vi "Initialize List Type.vi"(8 "error in (no error)":errorcluster, 11 "Numeric Data Type in":refnum<class "Numeric Data Type.lvclass">) -> (0 "error out":errorcluster, 3 "Numeric Data Type (dup)":refnum<class "Numeric Data Type.lvclass">)   [LabVIEW 2018, in "Numeric Data Type.lvclass"]
uses:
  Numeric Data Type.lvclass
  <vilib>/Utility/miscctls.llb/LVRowAndColumnUnsignedTypeDef.ctl
  Numeric Data Type.lvclass/Numeric Data Type.ctl
  Format Code Type List Enum.ctl
  Reference List Type.vi
  Reference Format Codes.vi
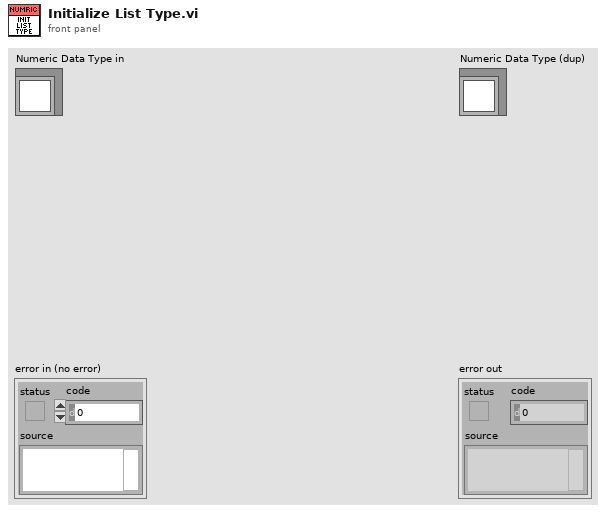
[diagram p1: front panel]
types:
  T1 = typedef "LVRowAndColumnUnsignedTypeDef.ctl" = cluster{"Row":u32, "Column":u32}
  T2 = typedef "Numeric Data Type.lvclass/Format Code Type List Enum.ctl" = enum16{"Numeric format codes", "Relative time format codes", "Absolute time format codes"}
  T3 = typedef "Numeric Data Type.lvclass/Time Info.ctl" = cluster{"Time Format":T4, "Numeric Format":T5, "Clock Type":T6, "Include Seconds?":bool, "Seconds Precision":i16, "Date Order":T7, "Date Format":T8, "Year Format":T9, "UTC":i16}
  T4 = typedef "Numeric Data Type.lvclass/Time Format.ctl" = enum16{"Custom time format", "System time format", "Time unused"}
  T5 = typedef "Numeric Data Type.lvclass/Numeric Format Enum.ctl" = enum16{"Floating Point Notation", "Scientific Notation", "Engineering Notation", "SI Notation", "<not used>", "Decimal", "Hexadecimal", "Octal", "Binary", "<not used 2>", "Absolute Time", "Relative Time"}
  T6 = typedef "Numeric Data Type.lvclass/Clock Type.ctl" = enum32{"12-Hour (AM/PM)", "24-Hour"}
  T7 = typedef "Numeric Data Type.lvclass/Date Order.ctl" = enum32{"M/D/Y", "D/M/Y", "Y/M/D"}
  T8 = typedef "Numeric Data Type.lvclass/Date Format.ctl" = enum16{"Custom date format", "System date format", "Date unused"}
  T9 = typedef "Numeric Data Type.lvclass/Year Format.ctl" = enum32{"No Year", "2-digit Year", "4-digit Year"}
  T10 = typedef "Numeric Data Type.lvclass/Numeric Info.ctl" = cluster{"Minimum Field Width":i32, "Digits of Precision":i32, "Numeric Format":T5, "Precision Type":T11, "Hide trailing zeros":bool, "exponent":bool, "just/pad":T12, "Modifiers":string}
  T11 = typedef "Numeric Data Type.lvclass/Precision Type.ctl" = enum16{"Digits of precision", "Significant digits"}
  T12 = typedef "Numeric Data Type.lvclass/Padding.ctl" = enum16{"Pad with spaces on left", "Pad with spaces on right", "Pad with zeros on left"}
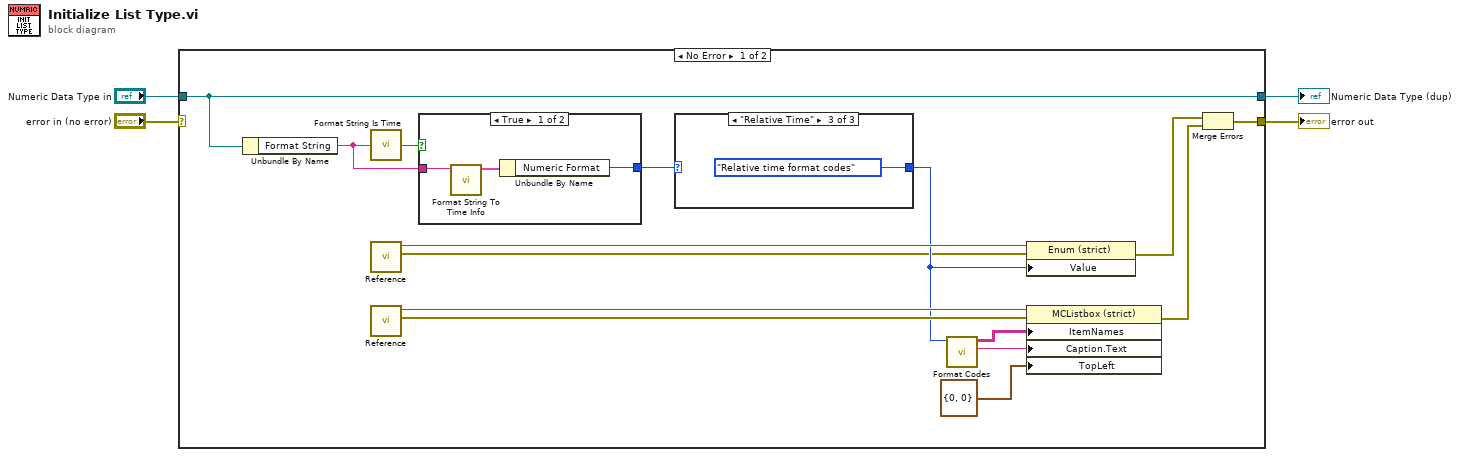
[diagram p0: block diagram]
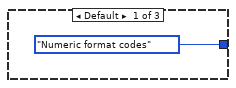
[diagram p2: hidden frame]
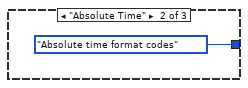
[diagram p3: hidden frame]
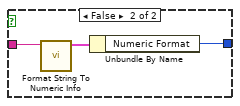
[diagram p4: hidden frame]
diagram:
  n1 = case shown="No Error" "error in (no error)" {
    selector: "error in (no error)" -> [_ w30]
    tunnel: [w8 w30] -> w3
    tunnel: [w19 w29] -> w1
    tunnel: "Numeric Data Type in" -> [w19 w29]
    frame No Error {
      n2 = Unbundle By Name(w19) -> ("Format String"=w16:string)
      n3 = call "Format String Is Time.vi"("Format String"=w16) -> ("Time?"=w17:bool)
      n4 = call-poly "Reference.vi"() -> ("error out"=w5:errorcluster, "List Type"=w10:refnum<vi>)  [unwired: 10 in]
      n5 = call-poly "Reference.vi"() -> ("error out"=w14:errorcluster, "Format Codes"=w15:refnum<vi>)  [unwired: 10 in]
      n6 = case shown="True" w17 {
        tunnel: w16 -> [w24 w27]
        tunnel: [w25 w28] -> w18
        frame True {
          n7 = call "Format String To Time Info.vi"("Format String"=w24) -> ("Time Info"=w23:T3)  [unwired: 10 in]
          n8 = Unbundle By Name(w23) -> ("Numeric Format"=w25:T5)
        }
        frame False {
          n9 = call "Format String To Numeric Info.vi"("Format String"=w27) -> ("Numeric Format & Precision Info"=w26:T10)  [unwired: 10 in]
          n10 = Unbundle By Name(w26) -> ("Numeric Format"=w28:T5)
        }
      }
      n11 = case shown="\"Relative Time\"" w18 {
        tunnel: [Format_Code_Type_List_Enum."Numeric format codes" ("Value") Format_Code_Type_List_Enum."Absolute time format codes" ("Value") Format_Code_Type_List_Enum."Relative time format codes" ("Value")] -> w6
        frame Default {
        }
        frame "Absolute Time" {
        }
        frame "Relative Time" {
        }
      }
      n12 = call "Format Codes.vi"("List type"=w6) -> ("Caption"=w12:string, "Item Names"=w13:string[][])  [unwired: 9 in]
      n13 = property class="Enum (strict)"(reference=w10, error in=w5, "Value"=w6) -> (error out=w9:errorcluster)  [unwired: 1 out]
      n14 = property on="Property Node" class="MCListbox (strict)"(reference=w15, error in=w14, "ItemNames"=w13, "Caption.Text"=w12, "TopLeft"=T1 {"Row"=0, "Column"=0} ("Top Left Visible Cell")) -> (error out=w7:errorcluster)  [unwired: 1 out]
      n15 = Merge Errors(w9, w7) -> (w8:errorcluster)
    }
    frame Error {
    }
  }
  "error out" <- w3
  "Numeric Data Type (dup)" <- w1
